vi "init.vi"(0 "virtual OSA":bool, 1 "virtual OSA model":T4, 2 "virtual source":T2={"OSA200"={"waveCenter (nm)"=1000.0, "FWHM (nm)"=0.001, "peakAmplitude"=0.001}, "OSA300"=enum."VIRTUAL_REDSTONE_SOURCE_UNKNOWN"} {"OSA200"."peakAmplitude" format="%#_6e"; "OSA200"."FWHM (nm)" format="%#_6e"; "OSA200"."waveCenter (nm)" format="%#_6e"}, 3 "buffer size interferogram (17E6)":i32=17000000 format="%^.0e", 4 "buffer size spectrum (1E6)":i32=1000000 format="%^.0e", 5 "error in (no error)":errorcluster, 6 "Graph Intrfrgrm":T5, 7 "peaks max nr (100)":u32=100, 8 "Graph Spectrum":T5, 9 "spectrIdx":u16, 11 "traces":T3={"nr interferogram (2)"=2, "nr spectrum (10)"=10}, 13 "FTSLV.dll path (dll\\util\\)":string) -> (14 "duplicate reference":refnum<class "OSA.lvclass">, 16 "spectrometer":string, 17 "waveNrMin":sgl format="%.2f", 18 "waveNrMax":sgl format="%.2f", 19 "error out":errorcluster)   [LabVIEW 2010, in "OSA.lvclass"]
doc: "Spectrometer selection and initialisation; for most applications the default values will be appropriate and need no connection, except for the graph references required when using distributed/TREE graph functions."
uses:
  OSA.lvclass
  private/graph_intensity.ctl
  _misc/Thorlabs_FTS_misc.llb/OSA_virtualModel.ctl
  _misc/Thorlabs_FTS_misc.llb/OSA_virtualSource_RS.ctl
  OSA20X_misc.lvlib
  _dll/LVLib/FTSLib.lvlib
panel:
  in  "plot zoom step factor":dbl=3.0 format="%.2f"
  out "#spectrometers":i32
  in  "duplicate reference 2":refnum<class "OSA.lvclass">
  in  "dialog":bool
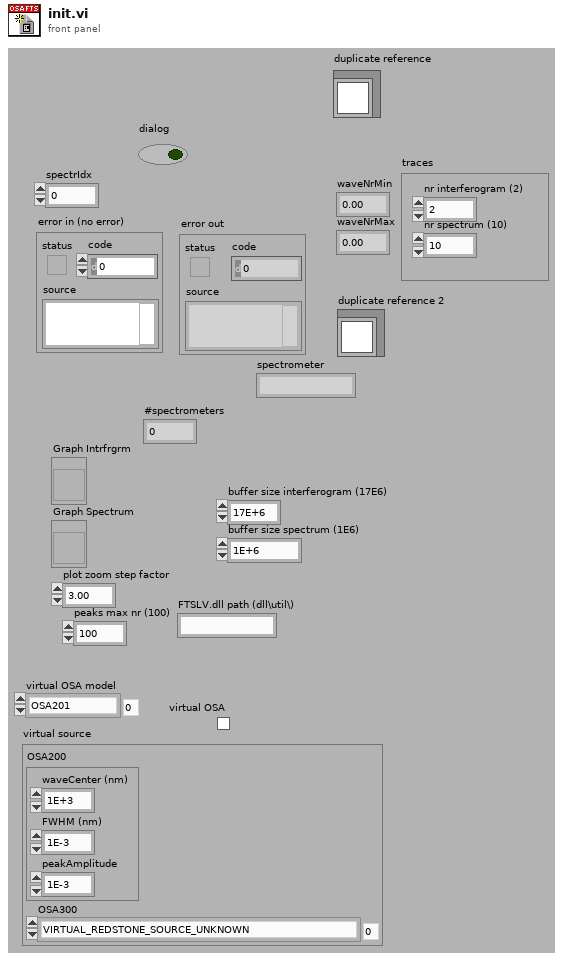
[diagram p1: front panel]
types:
  T1 = typedef "OSA20X_misc.lvlib/OSA_virtualSource_RS.ctl" = enum16{"VIRTUAL_REDSTONE_SOURCE_UNKNOWN", "VIRTUAL_REDSTONE_SOURCE_LLD_DFB_1530", "VIRTUAL_REDSTONE_SOURCE_SLD_1550nm", "VIRTUAL_REDSTONE_SOURCE_LASER_4600nm", "VIRTUAL_REDSTONE_SOURCE_BLACKBODY1500K", "VIRTUAL_REDSTONE_SOURCE_BLACKBODY1500K_H2O"}
  T2 = cluster{"OSA200":cluster{"waveCenter (nm)":dbl, "FWHM (nm)":dbl, "peakAmplitude":dbl}, "OSA300":T1}
  T3 = cluster{"nr interferogram (2)":i32, "nr spectrum (10)":i32}
  T4 = typedef "OSA20X_misc.lvlib/OSA_virtualModel.ctl" = enum16{"OSA201", "OSA201C", "OSA202", "OSA202C", "OSA203", "OSA203B", "OSA203C", "OSA205", "OSA205C", "REDSTONE301", "REDSTONE305"}
  T5 = typedef "OSA.lvclass/graph_intensity.ctl" = refnum<vi>
  T6 = enum16{"pressure", "temperature", "humidity", "all"}
  T7 = enum16{"add", "clear and add", "update", "remove", "none/read"}
  T8 = cluster{"waveCenter (nm)":dbl, "FWHM (nm)":dbl, "peakAmplitude":dbl}
  T9 = typedef "OSA.lvclass/OSA_series.ctl" = enum16{"OSA200", "OSA300", "UNKNOWN"}
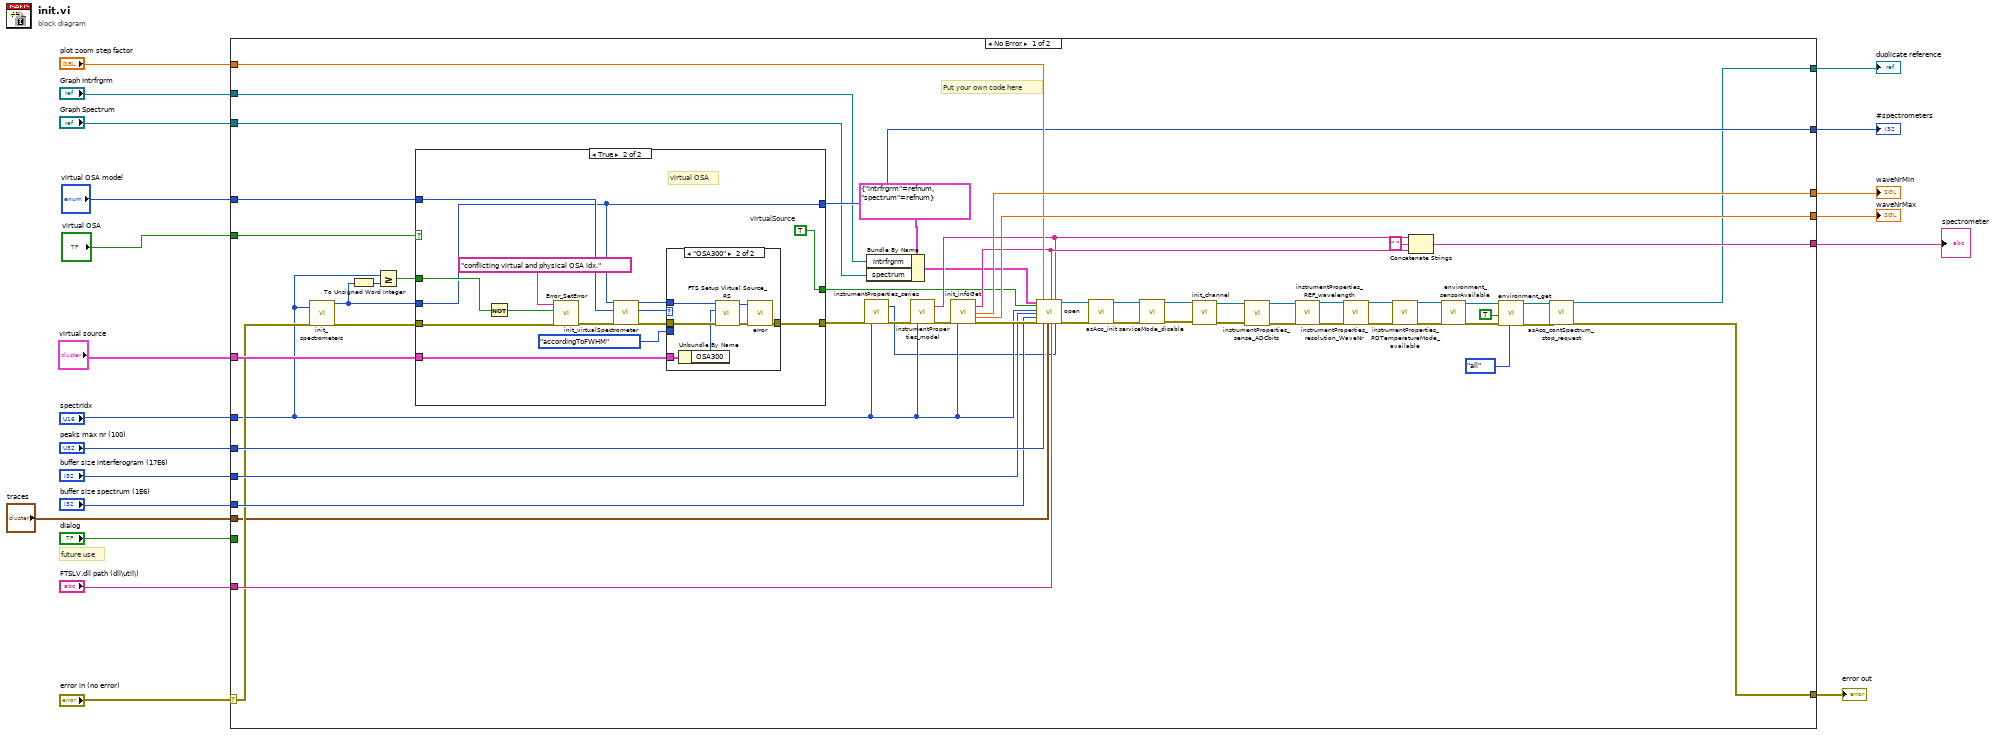
[diagram p0: block diagram]
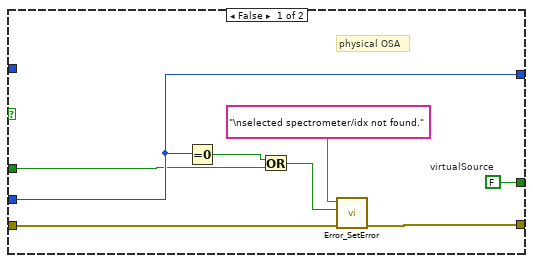
[diagram p2: hidden frame]
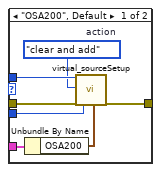
[diagram p3: hidden frame]
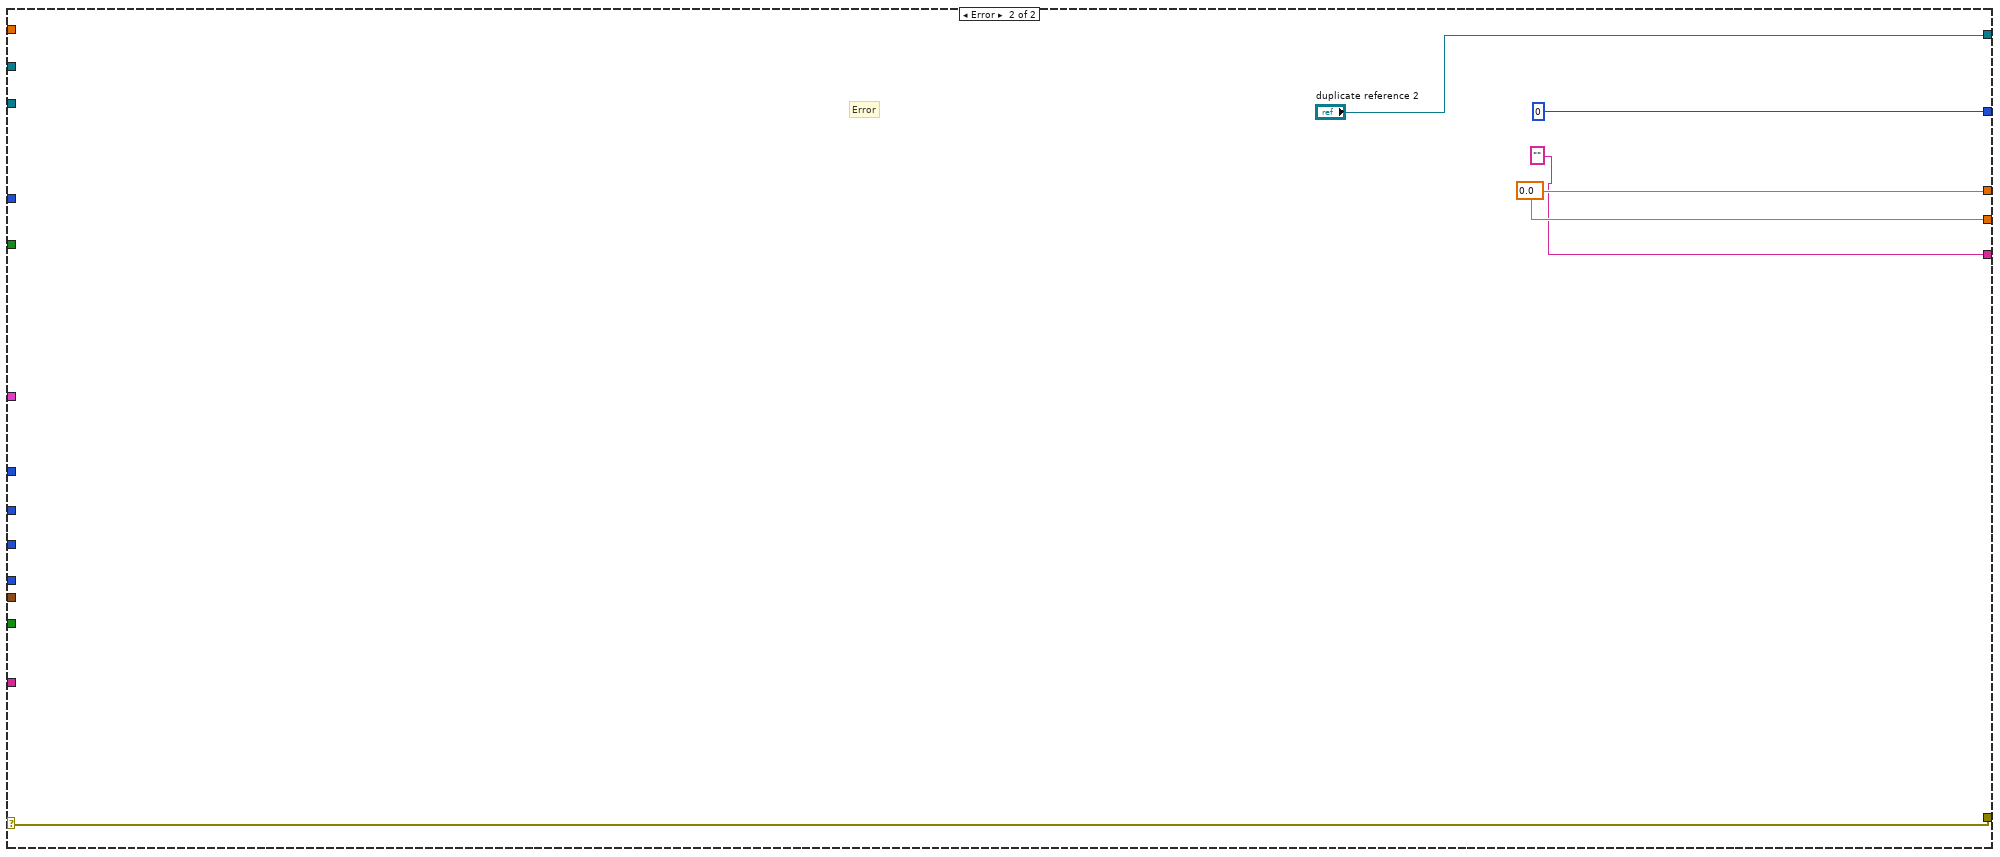
[diagram p4: hidden frame]
diagram:
  # "future use"
  n1 = case shown="No Error" "error in (no error)" {
    selector: "error in (no error)" -> [w58 w117]
    tunnel: [w44 w117] -> w19
    tunnel: [w45 "duplicate reference 2"] -> w18
    tunnel: "dialog" -> [_ _]
    tunnel: "spectrIdx" -> [w47 _]
    tunnel: [w75 w116] -> w15
    tunnel: [w74 w116] -> w14
    tunnel: [w56 0 ("#spectrometers")] -> w13
    tunnel: "Graph Intrfrgrm" -> [w39 _]
    tunnel: "Graph Spectrum" -> [w40 _]
    tunnel: "plot zoom step factor" -> [w73 _]
    tunnel: "peaks max nr (100)" -> [w72 _]
    tunnel: "FTSLV.dll path (dll\\util\\)" -> [w71 _]
    tunnel: "buffer size interferogram (17E6)" -> [w70 _]
    tunnel: "buffer size spectrum (1E6)" -> [w69 _]
    tunnel: [w64 "" ("serialNr")] -> w5
    tunnel: "virtual OSA" -> [w61 _]
    tunnel: "virtual OSA model" -> [w60 _]
    tunnel: "virtual source" -> [w59 _]
    tunnel: "traces" -> [w50 _]
    frame No Error {
      # "Put your own code here"
      n2 = call "init_spectrometers.vi"("spectrIdx"=w47, "error in (no error)"=w58) -> ("nr spectr found"=w54:i32, "error out"=w57:errorcluster)  [unwired: 16 in]
      n3 = To Unsigned Word Integer(number=w54) -> (unsigned 16bit integer=w55:u16)
      n4 = Greater Or Equal?(x=w47, y=w55) -> (x >= y?=w53:bool)
      n5 = case shown="True" w61 {
        tunnel: w57 -> [w78 w97]
        tunnel: [w83 w93] -> w49
        tunnel: w60 -> [_ w98]
        tunnel: w59 -> [_ w91]
        tunnel: w54 -> [w80 w87]
        tunnel: [w80 w87] -> w56
        tunnel: w53 -> [w79 w89]
        tunnel: [w77 w85] -> w25
        frame False {
          w77 = FALSE  # virtualSource
          # "physical OSA"
          n6 = Equal To 0?(x=w80) -> (x = 0?=w81:bool)
          n7 = Or(x=w81, y=w79) -> (x .or. y?=w82:bool)
          n8 = call "Error_SetError.vi"("error in"=w78, "status (true)"=w82, "source(\"\")"="\nselected spectrometer/idx not found." ("source(\"\")")) -> ("error out"=w83:errorcluster)  [unwired: 4 in]
        }
        frame True {
          w85 = TRUE  # virtualSource
          # "virtual OSA"
          n9 = Not(x=w89) -> (.not. x?=w88:bool)
          n10 = call "Error_SetError.vi"("error in"=w97, "status (true)"=w88, "source(\"\")"="conflicting virtual and physical OSA idx." ("source(\"\")")) -> ("error out"=w96:errorcluster)  [unwired: 4 in]
          n11 = call "init_virtualSpectrometer.vi"("idxSpectr"=w87, "model"=w98, "error in (no error)"=w96) -> ("idxSpectr copy"=w92:u16, "OSA series"=w86:enum16{"OSA200", "OSA300", "UNKNOWN"}, "error out"=w94:errorcluster)  [unwired: 14 in]
          n12 = case shown="\"OSA300\"" w86 {
            tunnel: w94 -> [w105 w112]
            tunnel: [w104 w106] -> w93
            tunnel: w92 -> [w103 w109]
            tunnel: w91 -> [w100 w111]
            tunnel: enum16{"monochromatic", "accordingToFWHM"}."accordingToFWHM" ("type") -> [w101 _]
            frame "OSA200", Default {
              w102 = T7."clear and add"  # action
              n13 = Unbundle By Name(w100) -> ("OSA200"=w99:T8)
              n14 = call "virtual_sourceSetup.vi"("idxSpectr"=w103, "action"=w102, "error in (no error)"=w105, "type"=w101, "source"=w99) -> ("error out"=w104:errorcluster)  [unwired: 10 in, 4 out]
            }
            frame "OSA300" {
              n15 = Unbundle By Name(w111) -> ("OSA300"=w110:T1)
              n16 = call "FTS Setup Virtual Source_RS.vi"("error in (no error)"=w112, "source type RS (LLD/DFB 1530nm)"=w110, "specIndex"=w109) -> ("error out"=w108:errorcluster, "function return"=w107:i32)  [unwired: 7 in]
              n17 = call "error.vi"("result code"=w107, "error in (no error)"=w108) -> ("error out"=w106:errorcluster)  [unwired: 15 in, 2 out]
            }
          }
        }
      }
      n18 = call "instrumentProperties_series.vi"("error in (no error)"=w49, "specIndex"=w47) -> ("OSA series"=w46:T9, "error out"=w48:errorcluster)  [unwired: 16 in]
      n19 = Bundle By Name(cluster=cluster{"intrfrgrm":T5, "spectrum":T5} {"intrfrgrm"=refnum, "spectrum"=refnum} ("graph"), "intrfrgrm"=w39, "spectrum"=w40) -> (w38:cluster{"intrfrgrm":T5, "spectrum":T5})
      n20 = call "instrumentProperties_model.vi"("error in (no error)"=w48, "spectrIdx"=w47) -> ("model"=w65:string, "error out"=w68:errorcluster)  [unwired: 16 in]
      n21 = call "init_infoGet.vi"("error in (no error)"=w68, "spectrIdx"=w47) -> ("serialNr"=w67:string, "waveNrMin"=w75:sgl, "waveNrMax"=w74:sgl, "error out"=w76:errorcluster)  [unwired: 14 in]
      n22 = call "open.vi"("graph"=w38, "virtualSource"=w25, "spectrIdx"=w47, "buffer size interferogram"=w70, "buffer size spectrum"=w69, "error in (no error)"=w76, "plot zoom step factor"=w73, "peaks max nr (100)"=w72, "traces"=w50, "spectrometer serial nr"=w67, "FTSLV.dll folder"=w71, "spectrometer model"=w65, "OSA series"=w46) -> ("duplicate reference"=w62:refnum<class "OSA.lvclass">, "error out"=w63:errorcluster)  [unwired: 5 in]
      n23 = call "asAcq_init.vi"("reference"=w62, "error in (no error)"=w63) -> ("duplicate reference"=w23:refnum<class "OSA.lvclass">, "error out"=w24:errorcluster)  [unwired: 16 in]
      n24 = call-dynamic "serviceMode_disable.vi"("error in (no error)"=w24, "Thorlabs_OSA_64 in"=w23) -> ("error out"=w21:errorcluster, "Thorlabs_OSA_64 out"=w22:refnum<class "OSA.lvclass">)  [unwired: 8 in]
      n25 = call-dynamic "init_channel.vi"("error in (no error)"=w21, "Thorlabs_OSA_64 in"=w22) -> ("error out"=w42:errorcluster, "Thorlabs_OSA_64 out"=w43:refnum<class "OSA.lvclass">)  [unwired: 8 in]
      n26 = call "instrumentProperties_sense_ADCbits.vi"("reference"=w43, "error in (no error)"=w42) -> ("duplicate reference"=w35:refnum<class "OSA.lvclass">, "error out"=w34:errorcluster)  [unwired: 15 in, 1 out]
      n27 = call "instrumentProperties_REF_wavelength.vi"("reference"=w35, "error in (no error)"=w34) -> ("duplicate reference"=w37:refnum<class "OSA.lvclass">, "error out"=w36:errorcluster)  [unwired: 15 in, 1 out]
      n28 = call "instrumentProperties_resolution_WaveNr.vi"("reference"=w37, "error in (no error)"=w36) -> ("duplicate reference"=w32:refnum<class "OSA.lvclass">, "error out"=w33:errorcluster)  [unwired: 15 in, 1 out]
      n29 = call-dynamic "instrumentProperties_PDTemperatureMode_available.vi"("reference"=w32, "error in (no error)"=w33) -> ("duplicate reference"=w30:refnum<class "OSA.lvclass">, "error out"=w31:errorcluster)  [unwired: 15 in, 1 out]
      n30 = Concatenate Strings(w65, " " ("string"), w67) -> (w64:string)
      n31 = call "environment_sensorAvailable.vi"("reference"=w30, "error in (no error)"=w31) -> ("duplicate reference"=w28:refnum<class "OSA.lvclass">, "error out"=w29:errorcluster)  [unwired: 13 in, 3 out]
      n32 = call "environment_get.vi"("reference"=w28, "read defaultValues"=TRUE, "error in (no error)"=w29, "parameter"=T6."all") -> ("duplicate reference"=w51:refnum<class "OSA.lvclass">, "error out"=w52:errorcluster)  [unwired: 8 in, 6 out]
      n33 = call "asAcq_contSpectrum_stop_request.vi"("reference"=w51, "error in (no error)"=w52) -> ("duplicate reference"=w45:refnum<class "OSA.lvclass">, "error out"=w44:errorcluster)  [unwired: 16 in]
    }
    frame Error {
      w116 = sgl 0.0 ("waveNrMin")
      # "Error"
    }
  }
  "error out" <- w19
  "duplicate reference" <- w18
  "waveNrMax" <- w14
  "waveNrMin" <- w15
  "#spectrometers" <- w13
  "spectrometer" <- w5
